vi "Update Limits.vi"(8 "error in":errorcluster, 9 "LowLim":dbl, 10 "HighLim":dbl, 11 "Limits Enabled?":bool) -> (0 "error out":errorcluster)   [LabVIEW 2014, in "Chart Module.lvlib"]
uses:
  Chart Module.lvlib
  Limits Argument--cluster.ctl
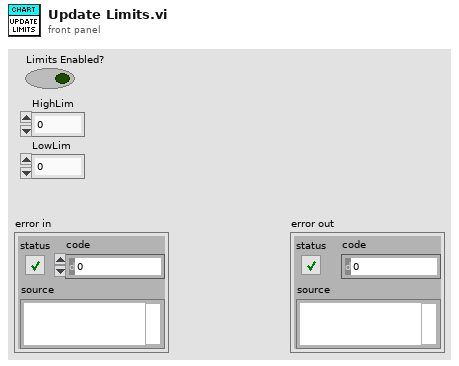
[diagram p1: front panel]
types:
  T1 = typedef "Chart Module.lvlib/Limits Argument--cluster.ctl" = cluster{"Enabled?":bool, "HighLim":dbl, "LowLim":dbl}
  T2 = typedef "Chart Module.lvlib/Request Events--cluster.ctl" = cluster{"Stop Module":refnum<user-event>, "Show Panel":refnum<user-event>, "Hide Panel":refnum<user-event>, "Update Limits":refnum<user-event>, "Send Value":refnum<user-event>, "Clear Chart":refnum<user-event>}
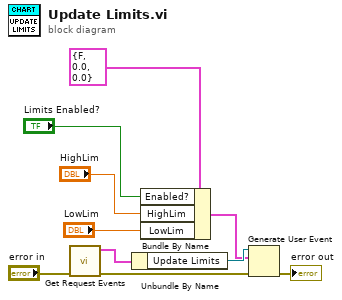
[diagram p0: block diagram]
diagram:
  n1 = call "Get Request Events.vi"("error in"="error in") -> ("error out"=w3:errorcluster, "Request Events"=w10:T2)  [unwired: 9 in]
  n2 = Unbundle By Name(w10) -> ("Update Limits"=w9:refnum<user-event>)
  n3 = Bundle By Name(cluster=T1 {"Enabled?"=FALSE, "HighLim"=0.0, "LowLim"=0.0} ("event data"), "Enabled?"="Limits Enabled?", "HighLim"="HighLim", "LowLim"="LowLim") -> (w7:T1)
  n4 = Generate User Event(user event=w9, event data cluster=w7, error in=w3) -> (error out=→"error out":errorcluster)  [unwired: 1 in, 1 out]
